vi "Write pathCalibrationFile.vi"(8 "error in (no error)":errorcluster, 10 "pathCalibrationFile":path, 11 "BME_DG_System in":refnum<class "BME_DG_System.lvclass">) -> (0 "error out":errorcluster, 3 "BME_DG_System out":refnum<class "BME_DG_System.lvclass">)   [LabVIEW 2009, in "BME_DG_System.lvclass"]
uses:
  BME_DG_System.lvclass
  BME_DG_System.lvclass/BME_DG_System.ctl
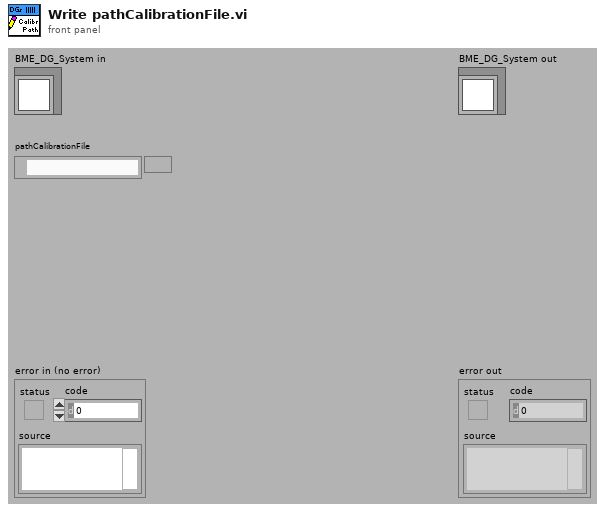
[diagram p1: front panel]
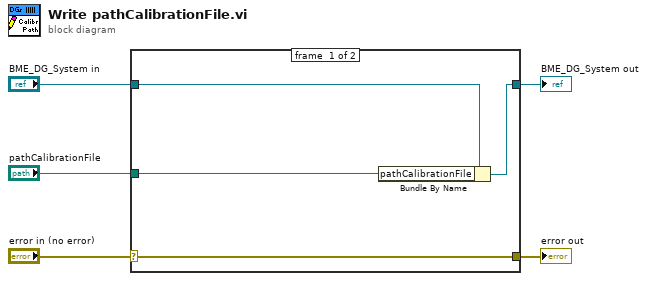
[diagram p0: block diagram]
diagram:
  n1 = case shown="No Error" "error in (no error)" {
    selector: "error in (no error)" -> [w9 w10]
    tunnel: [w9 w10] -> w4
    tunnel: [w7 w11] -> w2
    tunnel: "BME_DG_System in" -> [w8 w11]
    tunnel: "pathCalibrationFile" -> [w6 _]
    frame #0 {
      n2 = Bundle By Name(cluster=w8, "pathCalibrationFile"=w6) -> (w7:refnum<class "BME_DG_System.lvclass">)
    }
    frame #1 {
    }
  }
  "error out" <- w4
  "BME_DG_System out" <- w2
